vi "2021 Advent puzzle 03.vi"() -> ()   [LabVIEW 2021]
panel:
  out "Width":i32
  out "x*y":u64
  out "number 2":u32
  out "number":u32
  out "Array 2":bool[](array[boolean])
  out "column length":i32
  out "Array":i16[](array[numeric])
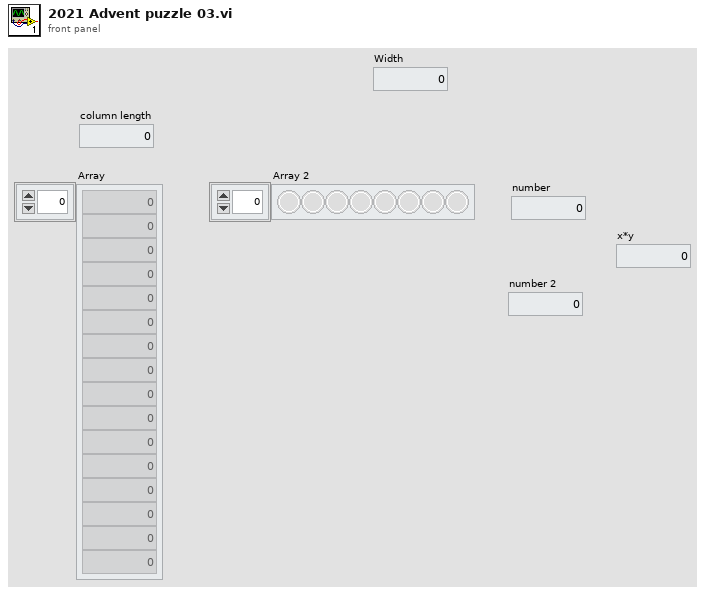
[diagram p1: front panel]
diagram:
  (unwired) "00100\n11110\n10110\n10111\n10101\n01111\n00111\n11100\n10000\n11001\n00010\n01010"
  w1 = "000001100010\n100111011010\n001100011001\n011010001010\n011010101011\n001001110101\n100110001101\n100010010011\n011110000110\n011000110110\n011111111110\n100111110011\n110000100101\n011010011111\n001010011101\n110110001010\n101111110101\n000010101101\n111010111110\n111110001110\n100110111011\n101011010101\n001001000101\n111101000100\n001100000010\n010001100101\n001010011111\n101010010100\n100001110011\n100000111010\n100101010101\n000000101000\n011010100011\n110100111110\n010010011000\n000101000010\n001100011100\n011101000000\n010110111010\n101101100100\n000000010011\n000101001111\n011011100111\n101111100101\n101001101011\n101100010100\n00..."
  # "calc number of 1s per original column\n(number > ((column length div 2 ))generates a true"
  # "determine the length of the line"
  n1 = Scan From String(format string="%s", input string=w1) -> (output 1=w15:string)  [unwired: 3 in, 3 out]
  n2 = Spreadsheet String To Array(delimiter (Tab)="\n", format string="%b", spreadsheet string=w1, array type (2D Dbl)=i32[] []) -> (array=w18:i32[])
  n3 = String Length(string=w15) -> (length=w14:i32)
  "Width" <- w14
  n4 = Array Size(array=w18) -> (size(s)=w12:i32)
  "column length" <- w12
  n5 = for {
    tunnel: w18 -> [w24] mode=indexing
    tunnel: [w23] -> w19 mode=indexing
    n6 = Number To Boolean Array(number=w24) -> (Boolean array=w23:bool[])
  }
  n7 = Transpose 2D Array(2D array=w19) -> (transposed array=w17:bool[][])
  n8 = Divide(x=w12, y=2) -> (x/y=w10:dbl)
  n9 = for {
    N: w14 -> [_]
    tunnel: w17 -> [w29] mode=indexing
    tunnel: [w26] -> w13 mode=indexing
    tunnel: w10 -> [w27]
    tunnel: [w25] -> w8 mode=indexing
    n10 = Boolean To (0,1)(Boolean=w29) -> (0, 1=w28:i16[])
    n11 = Add Array Elements(numeric array=w28) -> (sum=w26:i16)
    n12 = Greater?(x=w26, y=w27) -> (0:w25:bool)
  }
  "Array 2" <- w8
  n13 = Reverse 1D Array(array=w13) -> (reversed array=→"Array":i16[])
  n14 = Not(x=w8) -> (.not. x?=w7:bool[])
  n15 = Boolean Array To Number(Boolean array=w8) -> (number=w6:u32)
  "number" <- w6
  n16 = Boolean Array To Number(Boolean array=w7) -> (number=w5:u32)
  "number 2" <- w5
  n17 = To Unsigned Quad Integer(1:w6) -> (0:w3:u64)
  n18 = To Unsigned Quad Integer(1:w5) -> (0:w2:u64)
  n19 = Multiply(x=w3, y=w2) -> (x*y=→"x*y":u64)
